vi "niRFUtil TRC 2D DBL Array to Trace.vi"(7 "2D Real Array":sgl[][](array[numeric]) format="%.2f") -> (8 "Measurement Trace":T1 format="%.2f")   [LabVIEW 2015, in "niRFUtil.lvlib"]
uses:
  niRFUtil.lvlib
  Includes/niRFUtil INC Trace.ctl
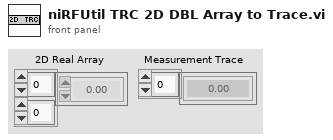
[diagram p1: front panel]
types:
  T1 = typedef "niRFUtil.lvlib/niRFUtil INC Trace.ctl" = sgl[]
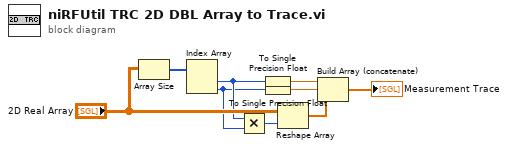
[diagram p0: block diagram]
diagram:
  n1 = Array Size(array="2D Real Array") -> (size(s)=w9:i32[])
  n2 = Index Array(array=w9) -> (element #1=w4:i32, element #2=w3:i32)  [unwired: 2 in]
  n3 = Multiply(x=w4, y=w3) -> (x*y=w2:i32)
  n4 = To Single Precision Float(number=w4) -> (single precision float=w7:sgl)
  n5 = To Single Precision Float(number=w3) -> (single precision float=w6:sgl)
  n6 = Reshape Array("2D Real Array", w2) -> (w5:sgl[])
  n7 = Build Array (concatenate)(w7, w6, w5) -> (→"Measurement Trace":sgl[])
